vi "DANTE test single.vi"() -> ()   [LabVIEW 2015]
panel:
  out "Waveform Graph":dbl[](graph)
  out "stats out":T1
  in  "Acquisition time [s]":dbl=10.0 min=1.0 max=1000.0
  out "DANTE configured":bool
  out "close [ms]":u32
  out "Acq [ms]":u32
  out "config [ms]":u32
  out "error out":errorcluster
  in  "DPP Configuration":T2={"reset_recovery_time"=300, "edge_peaking_time"=5, "flat_top"=5, "peaking_time"=25, "gain"=1.0, "max_risetime"=35.0, "fast_filter_thr"=100, "zero_peak_freq"=5.0, "inverted_input"=0, "base_offset"=0, "reset_threshold"=1000, "overflow_recovery"=0, "tail_coefficient"=0.0, "energy_filter_thr"=25, "energy_baseline_thr"=25, "max_peaking_time"=0, "edge_flat_top"=1, "time_constant"=0.0, "baseline_samples"=64, "other_param"=0}
  out "DANTE loaded":bool
  out "IP added":bool
  out "Library Initialized":bool
  in  "IP Address":string="10.96.0.110"
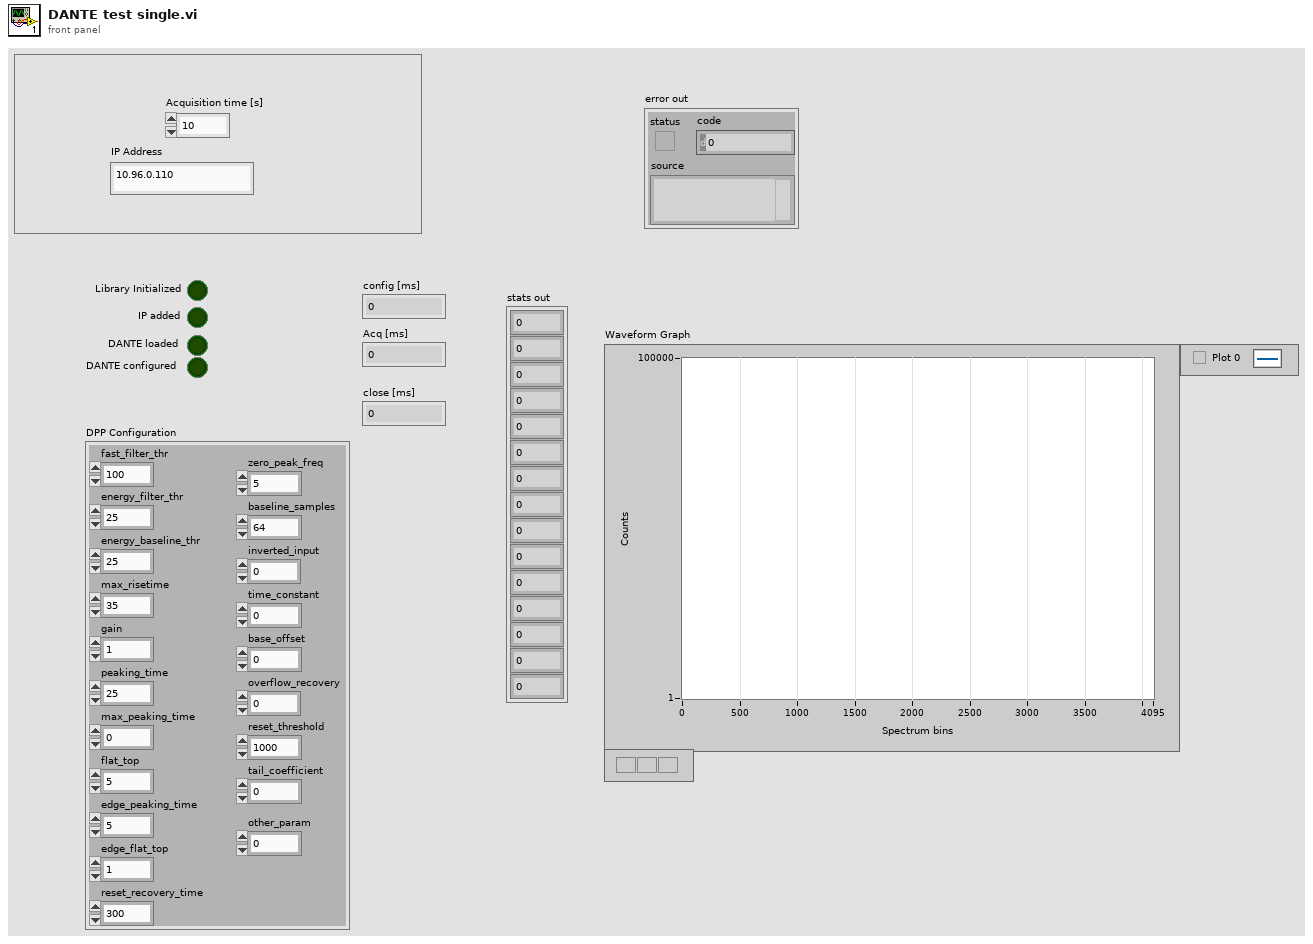
[diagram p1: front panel]
types:
  T1 = cluster{u64, u64, dbl, dbl, u32, u32, u32, u32, u32, u32, u32, u32, u32, u32, u32}
  T2 = cluster{"reset_recovery_time":u32, "edge_peaking_time":u32, "flat_top":u32, "peaking_time":u32, "gain":dbl, "max_risetime":dbl, "fast_filter_thr":u32, "zero_peak_freq":dbl, "inverted_input":u8, "base_offset":u32, "reset_threshold":u32, "overflow_recovery":u32, "tail_coefficient":dbl, "energy_filter_thr":u32, "energy_baseline_thr":u32, "max_peaking_time":u32, "edge_flat_top":u32, "time_constant":dbl, "baseline_samples":u32, "other_param":u32}
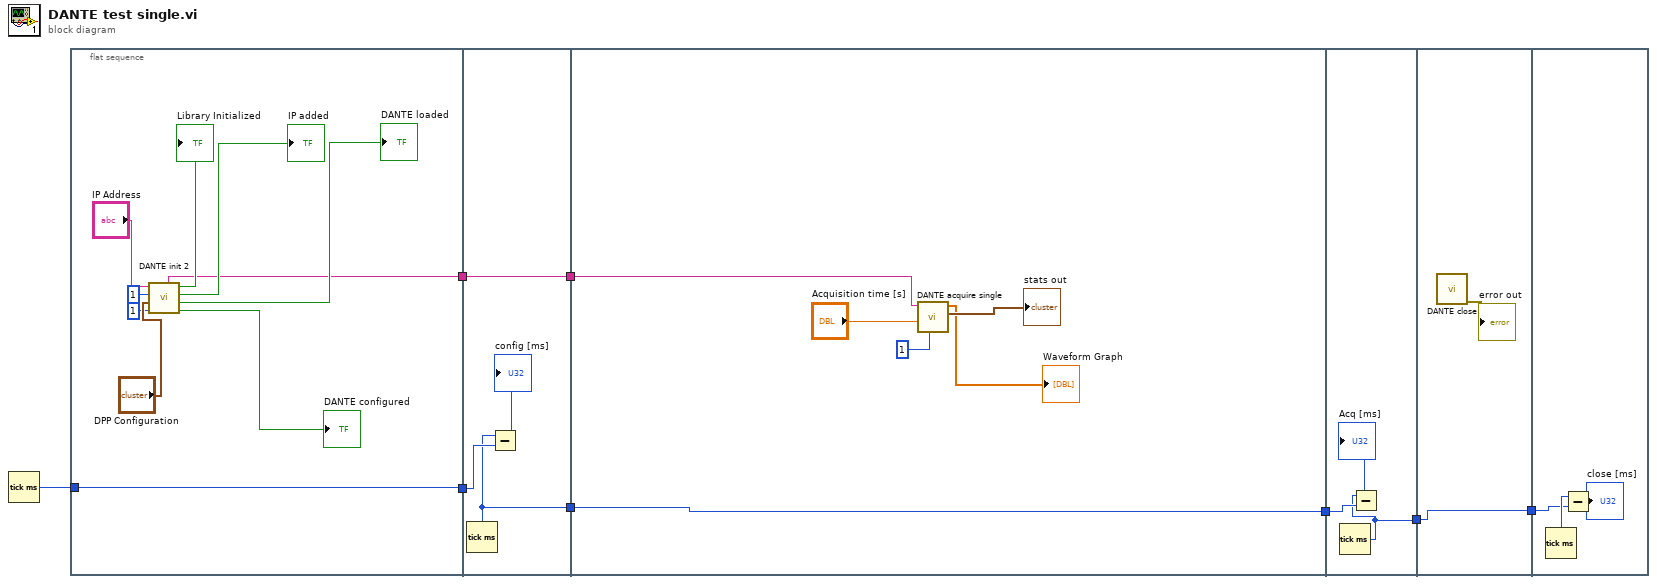
[diagram p0: block diagram]
diagram:
  n1 = Tick Count (ms)() -> (millisecond timer value=w8:u32)
  n2 = flat-sequence {
    tunnel: w8 -> [w17]
    tunnel: [w17] -> w7
    tunnel: [w9] -> w2
    tunnel: w7 -> [w22]
    tunnel: [w20] -> w6
    tunnel: w2 -> [w19]
    tunnel: [w19] -> w1
    tunnel: w6 -> [w28]
    tunnel: [w28] -> w5
    tunnel: w1 -> [w27]
    tunnel: w5 -> [w31]
    tunnel: [w29] -> w4
    tunnel: w4 -> [w32]
    tunnel: [w32] -> w3
    tunnel: w3 -> [w35]
    frame #0 {
      n3 = call "DANTE init 2.vi"("Boards to configure"=u8 1, "DPP Configuration"="DPP Configuration", "Number of boards in chain"=u8 1, "IP Address"="IP Address") -> ("DANTE configured"=→"DANTE configured":bool, "DANTE loaded"=→"DANTE loaded":bool, "IP added"=→"IP added":bool, "Library Initialized"=→"Library Initialized":bool, "identifier out"=w9:string)  [unwired: 3 in]
    }
    frame #1 {
      n4 = Tick Count (ms)() -> (millisecond timer value=w20:u32)
      n5 = Subtract(x=w20, y=w22) -> (x-y=→"config [ms]":u32)
    }
    frame #2 {
      n6 = call "DANTE acquire single.vi"("Number of boards in chain"=u8 1, "Acquisition time [s]"="Acquisition time [s]", "identifier out"=w27) -> ("stats out"=→"stats out":T1, "single spectrum"=→"Waveform Graph":dbl[])  [unwired: 7 in]
    }
    frame #3 {
      n7 = Tick Count (ms)() -> (millisecond timer value=w29:u32)
      n8 = Subtract(x=w29, y=w31) -> (x-y=→"Acq [ms]":u32)
    }
    frame #4 {
      n9 = call "DANTE close.vi"() -> ("error out"=→"error out":errorcluster)  [unwired: 9 in, 2 out]
    }
    frame #5 {
      n10 = Tick Count (ms)() -> (millisecond timer value=w36:u32)
      n11 = Subtract(x=w36, y=w35) -> (x-y=→"close [ms]":u32)
    }
  }
